vi "Mark Selected Error As Read.vi"(1 "MCL Row Index (display drder)":i32, 2 "Handled Errors (display order)":T1[](array[typedef])) -> (0 "Handled Errors (display order)":T1[](array[typedef]))   [LabVIEW 2023, in "Error Manager.lvlib"]
doc: "This VI updates the \"Read-Unread Status\" of a handled error to Read. This marks the Handled Error as read."
uses:
  Error Manager.lvlib
  Handled Error (cluster).ctl
  Read-Unread Status (enum).ctl
panel:
  # "Development\nControls or indicators that are useful for development or testing, but which are not outputs of the VI."
  # "Input\nInputs to the VI"
  # "Output\nOutputs of the VI"
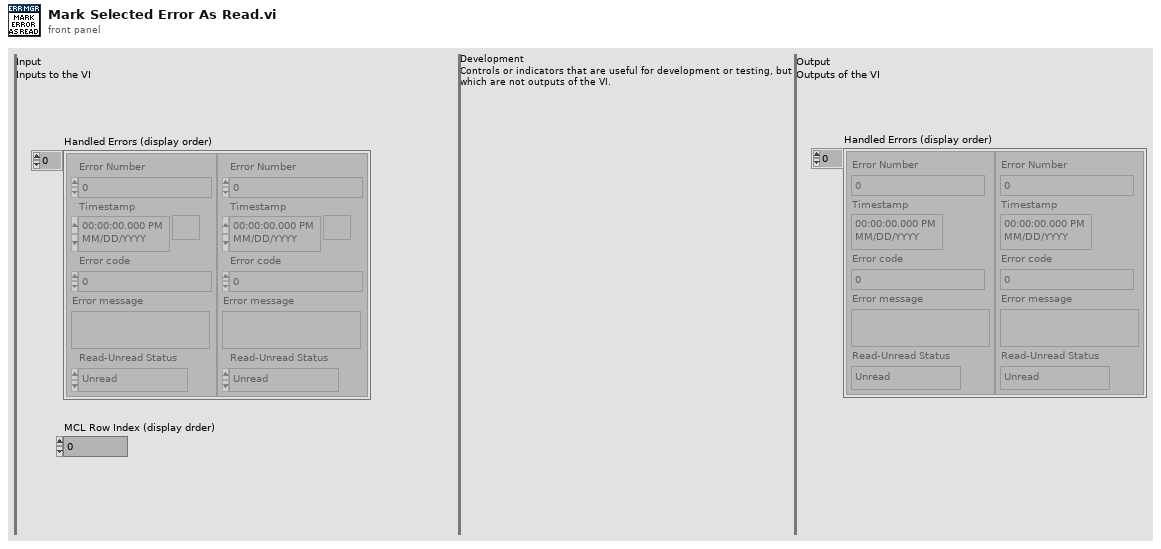
[diagram p1: front panel]
types:
  T1 = typedef "Error Manager.lvlib/Handled Error (cluster).ctl" = cluster{"Error Number":i32, "Timestamp":timestamp, "Error code":i32, "Error message":string, "Read-Unread Status":T2}
  T2 = typedef "Error Manager.lvlib/Read-Unread Status (enum).ctl" = enum16{"Unread", "Read"}
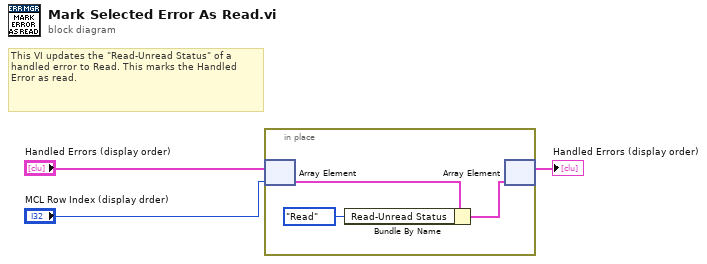
[diagram p0: block diagram]
diagram:
  # "This VI updates the \"Read-Unread Status\" of a handled error to Read. This marks the Handled Error as read."
  n1 = in-place {
    n2 = in-place-array #1("Handled Errors (display order)", "MCL Row Index (display drder)") -> (w5:T1)
    n3 = Bundle By Name(cluster=w5, "Read-Unread Status"=Read-Unread_Status_(enum)."Read") -> (w4:T1)
    n4 = in-place-array #1(w4) -> (→"Handled Errors (display order)":T1[])  [unwired: 1 out]
  }
